vi "Generate File Test Vector Table.vi"(8 "error in (no error)":errorcluster, 11 "LUnit Test Vector in":refnum<class "LUnit Test Vector.lvclass">) -> (0 "error out":errorcluster, 2 "Test Vector Table":string, 3 "LUnit Test Vector out":refnum<class "LUnit Test Vector.lvclass">)   [LabVIEW 2020, in "LUnit Test Vector.lvclass"]
uses:
  LUnit Test Vector.lvclass
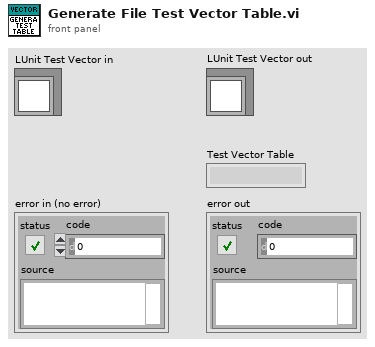
[diagram p1: front panel]
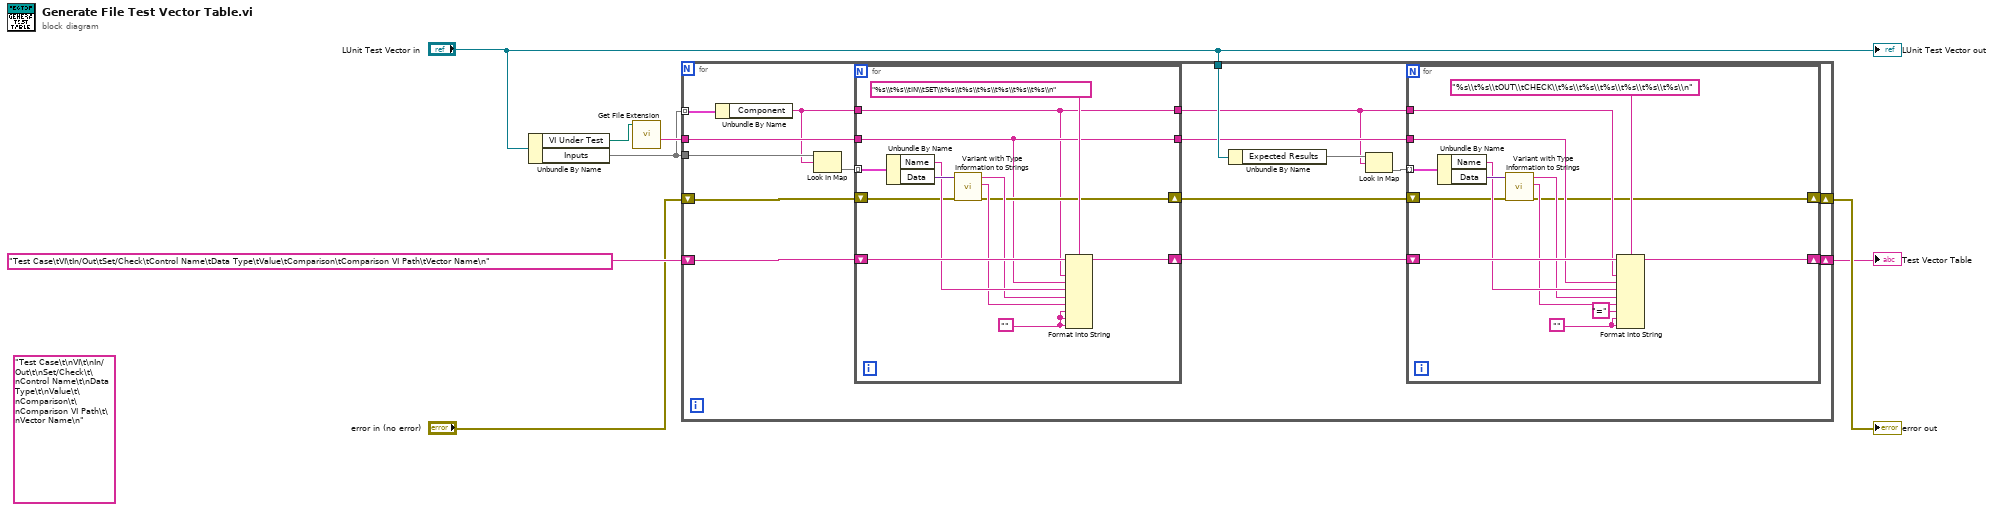
[diagram p0: block diagram]
diagram:
  (unwired) "Test Case\t\nVI\t\nIn/Out\t\nSet/Check\t\nControl Name\t\nData Type\t\nValue\t\nComparison\t\nComparison VI Path\t\nVector Name\n"
  n1 = Unbundle By Name("LUnit Test Vector in") -> ("VI Under Test"=w7:path, "Inputs"=w1:map{string, map{string, variant}})
  n2 = call <vilib>:"Get File Extension.vi"("file"=w7) -> ("filename without extension"=w6:string)  [unwired: 6 in, 4 out]
  n3 = for {
    tunnel: w6 -> [w23]
    tunnel: w1 -> [w22] mode=indexing
    tunnel: "LUnit Test Vector in" -> [w19]
    shift-right: [w15] -> w2
    shift-left: "Test Case\tVI\tIn/Out\tSet/Check\tControl Name\tData Type\tValue\tComparison\tComparison VI Path\tVector Name\n" -> [w24]
    shift-right: [w16] -> w3
    shift-left: "error in (no error)" -> [w21]
    tunnel: w1 -> [w12]
    n4 = Unbundle By Name(w22) -> ("Component"=w10:string)
    n5 = Look In Map(map=w12, key=w10) -> (value=w13:map{string, variant})  [unwired: 1 in, 1 out]
    n6 = for {
      shift-right: [w35] -> w17
      shift-left: w24 -> [w36]
      tunnel: w13 -> [w34] mode=indexing
      tunnel: w10 -> [w25]
      tunnel: w23 -> [w26]
      shift-right: [w28] -> w18
      shift-left: w21 -> [w29]
      tunnel: [w26] -> w11
      tunnel: [w25] -> w9
      w27 = ""
      n7 = Unbundle By Name(w34) -> ("Name"=w32:string, "Data"=w33:variant)
      n8 = call "Variant with Type Information to Strings.vi"("error in (no error)"=w29, "Variant"=w33) -> ("error out"=w28:errorcluster, "Data"=w30:string, "Datatype"=w31:string)  [unwired: 7 in]
      n9 = Format Into String(format string="%s\\t%s\\tIN\\tSET\\t%s\\t%s\\t%s\\t%s\\t%s\\t%s\\n", initial string=w36, w25, w26, w32, w31, w30, w27, w27, w27) -> (resulting string=w35:string)  [unwired: 1 in, 1 out]
    }
    n10 = Unbundle By Name(w19) -> ("Expected Results"=w20:map{string, map{string, variant}})
    n11 = Look In Map(map=w20, key=w9) -> (value=w14:map{string, variant})  [unwired: 1 in, 1 out]
    n12 = for {
      shift-right: [w49] -> w15
      shift-left: w17 -> [w50]
      tunnel: w14 -> [w46] mode=indexing
      tunnel: w9 -> [w48]
      tunnel: w11 -> [w47]
      shift-right: [w39] -> w16
      shift-left: w18 -> [w40]
      w38 = ""
      n13 = Unbundle By Name(w46) -> ("Name"=w44:string, "Data"=w45:variant)
      n14 = call "Variant with Type Information to Strings.vi"("error in (no error)"=w40, "Variant"=w45) -> ("error out"=w39:errorcluster, "Data"=w42:string, "Datatype"=w43:string)  [unwired: 7 in]
      n15 = Format Into String(format string="%s\\t%s\\tOUT\\tCHECK\\t%s\\t%s\\t%s\\t%s\\t%s\\t%s\\n", initial string=w50, w48, w47, w44, w43, w42, "=" ("input 6"), w38, w38) -> (resulting string=w49:string)  [unwired: 1 in, 1 out]
    }
  }
  "Test Vector Table" <- w2
  "error out" <- w3
  "LUnit Test Vector out" <- "LUnit Test Vector in"
